vi "Swerve Drive.vi"(0 "X":dbl, 1 "Rot. Point X":dbl, 3 "Rot. Point Y":dbl, 5 "Y":dbl, 7 "Z":dbl, 11 "Error In":errorcluster, 12 "Robot Centric?":bool=TRUE, 13 "Autonomous?":bool, 14 "Yaw":dbl) -> (4 "Front Left Output":dbl, 6 "Front Right Output":dbl, 8 "Back Left Output":dbl, 10 "Back Right Output":dbl, 15 "Error Out":errorcluster)   [LabVIEW 2016]
uses:
  <vilib>/Rock Robotics/Network Tables/NT Read Number.vi
  <vilib>/Rock Robotics/Network Tables/NT Write Numeric Array.vi
panel:
  in  "Robot Length":dbl=33.5
  in  "Robot Width":dbl=28.5
  # "Swerve Drive Teleoperated Control\nFRC Team 34"
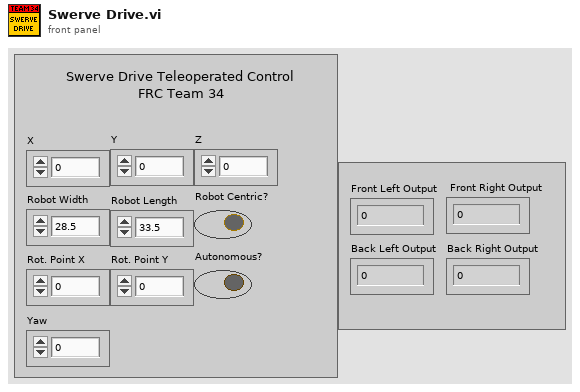
[diagram p1: front panel]
types:
  T1 = enum16{"Front Left", "Front Right", "Back Left", "Back Right"}
  T2 = typedef "WPI_MotorControlDeviceRef.ctl" = cluster{"DeviceStatus":errorcluster, "Type":T3, "PWM":cluster{"PWM Channel":T4, "DeadBand":T5}, "CAN":cluster{"Device Number":u8, "SetOutput VI Ref":variant, "GetOutput VI Ref":variant, "Enable VI Ref":variant, "Disable VI Ref":variant, "Data":variant}, "Invert":bool}
  T3 = typedef "WPI_MotorControlType.ctl" = enum16{"PWM", "CAN"}
  T4 = typedef "FPGA_DIOPWMChannel.ctl" = enum8{"PWM 0", "PWM 1", "PWM 2", "PWM 3", "PWM 4", "PWM 5", "PWM 6", "PWM 7", "PWM 8", "PWM 9", "PWM MXP 0", "PWM MXP 1", "PWM MXP 2", "PWM MXP 3", "PWM MXP 4", "PWM MXP 5", "PWM MXP 6", "PWM MXP 7", "PWM MXP 8", "PWM MXP 9", "Invalid"}
  T5 = typedef "WPI_PWMDeadband.ctl" = cluster{"Name":string, "maxPositivePwm":i32, "minPositivePwm":i32, "centerPwm":i32, "maxNegativePwm":i32, "minNegativePwm":i32, "angularRange":u16}
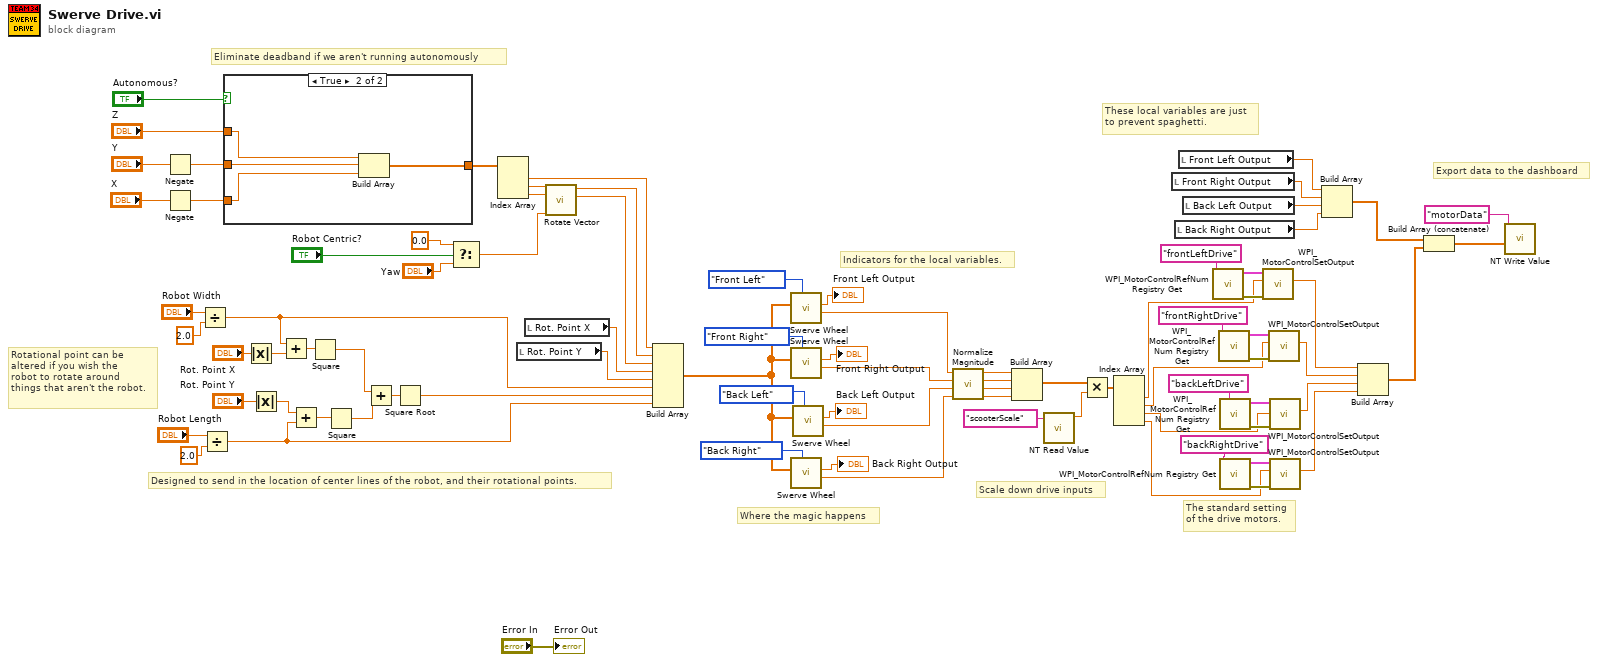
[diagram p0: block diagram]
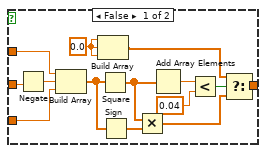
[diagram p2: hidden frame]
diagram:
  # "Indicators for the local variables."
  # "Rotational point can be \naltered if you wish the \nrobot to rotate around \nthings that aren't the robot."
  # "Scale down drive inputs"
  # "Eliminate deadband if we aren't running autonomously"
  # "These local variables are just \nto prevent spaghetti."
  # "Export data to the dashboard"
  # "Where the magic happens"
  # "The standard setting\nof the drive motors."
  # "Designed to send in the location of center lines of the robot, and their rotational points."
  n1 = Negate(x="Y") -> (-x=w2:dbl)
  n2 = Negate(x="X") -> (-x=w1:dbl)
  n3 = Divide(x="Robot Width", y=2.0) -> (x/y=w57:dbl)
  n4 = Divide(x="Robot Length", y=2.0) -> (x/y=w55:dbl)
  n5 = case shown="True" "Autonomous?" {
    tunnel: w2 -> [w88 w101]
    tunnel: [w87 w99] -> w83
    tunnel: "Z" -> [w86 w102]
    tunnel: w1 -> [w85 w100]
    frame False {
      w94 = 0.0 ("element")
      n6 = Negate(x=w88) -> (-x=w90:dbl)
      n7 = Build Array(w86, w90, w85) -> (w93:dbl[])
      n8 = Build Array(w94, w94, w94) -> (w95:dbl[])
      n9 = Square(x=w93) -> (x^2=w91:dbl[])
      n10 = Sign(1:w93) -> (0:w92:dbl[])
      n11 = Multiply(x=w91, y=w92) -> (x*y=w89:dbl[])
      n12 = Add Array Elements(numeric array=w91) -> (sum=w98:dbl)
      n13 = Less?(x=w98, y=0.04 ("x")) -> (x < y?=w96:bool)
      n14 = Select(t=w95, s=w96, f=w89) -> (s? t:f=w87:dbl[])
    }
    frame True {
      n15 = Build Array(w102, w101, w100) -> (w99:dbl[])
    }
  }
  n16 = Absolute Value(x="Rot. Point X") -> (abs(x)=w69:dbl)
  n17 = Absolute Value(x="Rot. Point Y") -> (abs(x)=w66:dbl)
  n18 = Add(x=w57, y=w69) -> (x+y=w68:dbl)
  n19 = Add(x=w66, y=w55) -> (x+y=w67:dbl)
  n20 = Square(x=w68) -> (x^2=w64:dbl)
  n21 = Square(x=w67) -> (x^2=w65:dbl)
  n22 = Add(x=w64, y=w65) -> (x+y=w63:dbl)
  n23 = Square Root(x=w63) -> (sqrt(x)=w56:dbl)
  n24 = Select(t=0.0, s="Robot Centric?", f="Yaw") -> (s? t:f=w76:dbl)
  n25 = Index Array(array=w83) -> (element #1=w62:dbl, element #2=w78:dbl, element #3=w77:dbl)  [unwired: 3 in]
  n26 = local read "Rot. Point Y"() -> (w58:dbl)
  n27 = local read "Rot. Point X"() -> (w59:dbl)
  n28 = call "Rotate Vector.vi"("Angle"=w76, "X"=w77, "Y"=w78) -> ("X'"=w60:dbl, "Y'"=w61:dbl)  [unwired: 7 in]
  n29 = Build Array(w62, w61, w60, w59, w58, w57, w56, w55) -> (w54:dbl[])
  n30 = call "Swerve Wheel.vi"("Wheel"=T1."Front Left", "Inputs"=w54) -> ("Speed"=w49:dbl, "Motor Output"=→"Front Left Output":dbl)  [unwired: 8 in]
  n31 = call "Swerve Wheel.vi"("Wheel"=T1."Front Right", "Inputs"=w54) -> ("Speed"=w48:dbl, "Motor Output"=→"Front Right Output":dbl)  [unwired: 8 in]
  n32 = call "Swerve Wheel.vi"("Wheel"=T1."Back Right", "Inputs"=w54) -> ("Speed"=w46:dbl, "Motor Output"=→"Back Right Output":dbl)  [unwired: 8 in]
  n33 = call "Swerve Wheel.vi"("Wheel"=T1."Back Left", "Inputs"=w54) -> ("Speed"=w47:dbl, "Motor Output"=→"Back Left Output":dbl)  [unwired: 8 in]
  n34 = call "Normalize Magnitude.vi"("D"=w46, "C"=w47, "B"=w48, "A"=w49) -> ("D'"=w22:dbl, "C'"=w23:dbl, "B'"=w24:dbl, "A'"=w25:dbl)  [unwired: 4 in]
  n35 = Build Array(w25, w24, w23, w22) -> (w21:dbl[])
  n36 = call-poly <vilib>:"NT Read Value.vi"("Name"="scooterScale") -> ("Numeric"=w19:dbl)  [unwired: 9 in, 1 out]
  n37 = Multiply(x=w21, y=w19) -> (x*y=w18:dbl[])
  n38 = Index Array(array=w18) -> (element #1=w17:dbl, element #2=w16:dbl, element #3=w15:dbl, element #4=w14:dbl)  [unwired: 4 in]
  n39 = local read "Front Right Output"() -> (w7:dbl)
  n40 = local read "Back Right Output"() -> (w5:dbl)
  n41 = local read "Front Left Output"() -> (w8:dbl)
  n42 = local read "Back Left Output"() -> (w6:dbl)
  n43 = call <vilib>:"WPI_MotorControlRefNum Registry Get.vi"("refnum name"="frontLeftDrive") -> ("error out"=w44:errorcluster, "MotorControlDevRef"=w43:T2)  [unwired: 9 in]
  n44 = call <vilib>:"WPI_MotorControlRefNum Registry Get.vi"("refnum name"="frontRightDrive") -> ("error out"=w39:errorcluster, "MotorControlDevRef"=w42:T2)  [unwired: 9 in]
  n45 = call <vilib>:"WPI_MotorControlRefNum Registry Get.vi"("refnum name"="backLeftDrive") -> ("error out"=w38:errorcluster, "MotorControlDevRef"=w40:T2)  [unwired: 9 in]
  n46 = call <vilib>:"WPI_MotorControlRefNum Registry Get.vi"("refnum name"="backRightDrive") -> ("error out"=w36:errorcluster, "MotorControlDevRef"=w35:T2)  [unwired: 9 in]
  n47 = call <vilib>:"WPI_MotorControlSetOutput.vi"("error in (no error)"=w44, "Output"=w17, "MotorControlDevRef"=w43) -> ("Motor Output"=w33:dbl)  [unwired: 6 in, 2 out]
  n48 = call <vilib>:"WPI_MotorControlSetOutput.vi"("error in (no error)"=w39, "Output"=w16, "MotorControlDevRef"=w42) -> ("Motor Output"=w32:dbl)  [unwired: 6 in, 2 out]
  n49 = call <vilib>:"WPI_MotorControlSetOutput.vi"("error in (no error)"=w38, "Output"=w15, "MotorControlDevRef"=w40) -> ("Motor Output"=w31:dbl)  [unwired: 6 in, 2 out]
  n50 = call <vilib>:"WPI_MotorControlSetOutput.vi"("error in (no error)"=w36, "Output"=w14, "MotorControlDevRef"=w35) -> ("Motor Output"=w30:dbl)  [unwired: 6 in, 2 out]
  n51 = Build Array(w8, w7, w6, w5) -> (w28:dbl[])
  n52 = Build Array(w33, w32, w31, w30) -> (w29:dbl[])
  n53 = Build Array (concatenate)(w28, w29) -> (w27:dbl[])
  n54 = call-poly <vilib>:"NT Write Value.vi"("Numeric Array"=w27, "Name"="motorData") -> ()  [unwired: 9 in, 1 out]
  "Error Out" <- "Error In"
